vi "reshape array (AIM-1553-frames).vi"(10 "index requested":i32=2, 11 "map array in":map{string, map{string, T1}}[](array[numeric])) -> (3 "map array out":map{string, map{string, T1}}[](array[numeric]))   [LabVIEW 2020]
uses:
  1553/_controls/1553_minorFrames.ctl
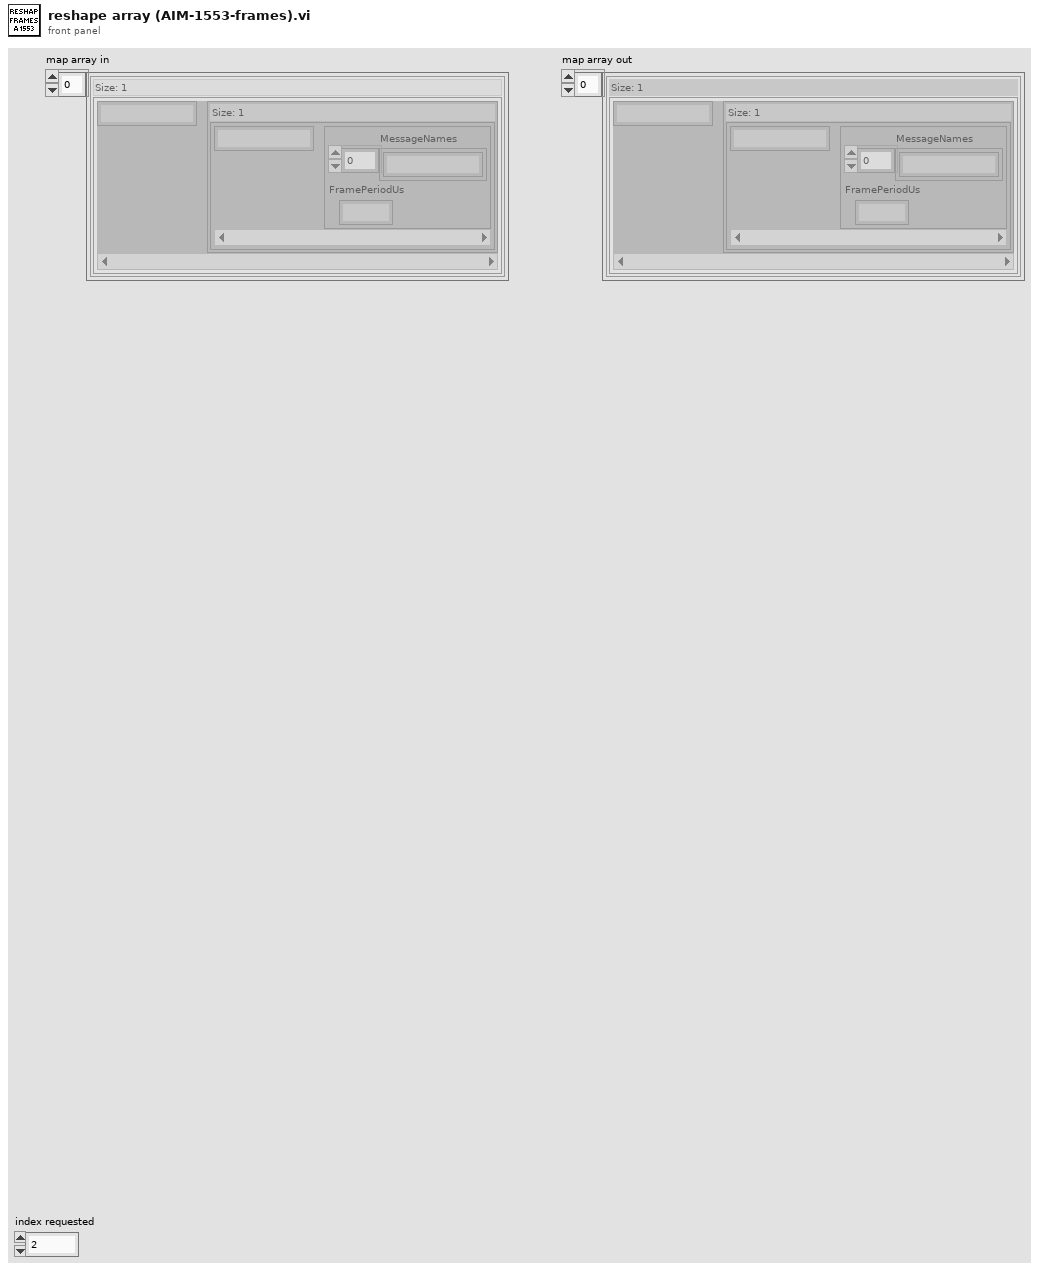
[diagram p1: front panel]
types:
  T1 = typedef "1553_minorFrames.ctl" = cluster{"MessageNames":string[], "FramePeriodUs":i32}
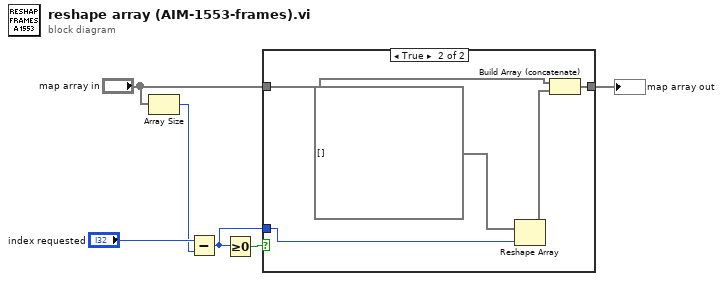
[diagram p0: block diagram]
diagram:
  n1 = Array Size(array="map array in") -> (size(s)=w5:i32)
  n2 = Subtract(x="index requested", y=w5) -> (x-y=w3:i32)
  n3 = Greater Or Equal To 0?(x=w3) -> (x >= 0?=w4:bool)
  n4 = case shown="True" w4 {
    tunnel: w3 -> [_ w12]
    tunnel: "map array in" -> [w7 w10]
    tunnel: [w7 w9] -> w1
    frame False {
    }
    frame True {
      n5 = Reshape Array(map{string, map{string, T1}}[] [] ("map array in 2"), w12) -> (w11:map{string, map{string, T1}}[])
      n6 = Build Array (concatenate)(w10, w11) -> (w9:map{string, map{string, T1}}[])
    }
  }
  "map array out" <- w1
